vi "squre root.vi"() -> ()   [LabVIEW 2016]
panel:
  out "Squre root Value":dbl
  in  "Number":dbl
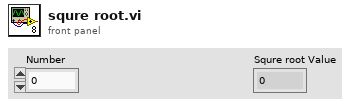
[diagram p1: front panel]
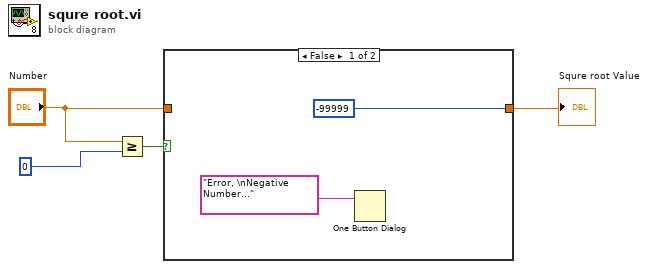
[diagram p0: block diagram]
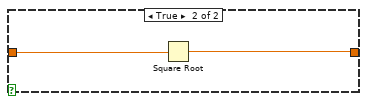
[diagram p2: hidden frame]
diagram:
  n1 = Greater Or Equal?(x="Number", y=0) -> (x >= y?=w3:bool)
  n2 = case shown="False" w3 {
    tunnel: [-99999 w8] -> w2
    tunnel: "Number" -> [_ w7]
    frame False {
      n3 = One Button Dialog(message="Error, \nNegative Number...") -> ()  [unwired: 1 in, 1 out]
    }
    frame True {
      n4 = Square Root(x=w7) -> (sqrt(x)=w8:dbl)
    }
  }
  "Squre root Value" <- w2
